vi "Memory.Pointer.Write.Safe.1D.U64.vi"(8 "error in (no error)":errorcluster, 9 "count":u64 format="%d elements", 10 "buffer in":u64[](array[numeric]), 11 "pointer in":refnum<class "Memory.Pointer.lvclass">) -> (0 "error out":errorcluster, 2 "buffer out":u64[](array[numeric]), 3 "pointer out":refnum<class "Memory.Pointer.lvclass">)   [LabVIEW 2016, in "Memory Manager.lvlib" / "Memory.Pointer.lvclass"]
doc: "Writes <b>count</b> elements from the provided <b>buffer</b> to the address specified by <b>pointer</b>.\n\n<b>Note:</b> This VI is <b>safe</b>.\n\nSafe means that this function evaluates the size parameter of <b>pointer</b> to ensure that is inbounds of allocated memory before peforming a memory read/write. Reading/writing more data to a pointer than it has allocated can corrupt or crash LabVIEW."
uses:
  Memory.Pointer.lvclass
  Memory.Pointer.lvclass/Memory.Pointer.ctl
  Accessors/Get Address.vi
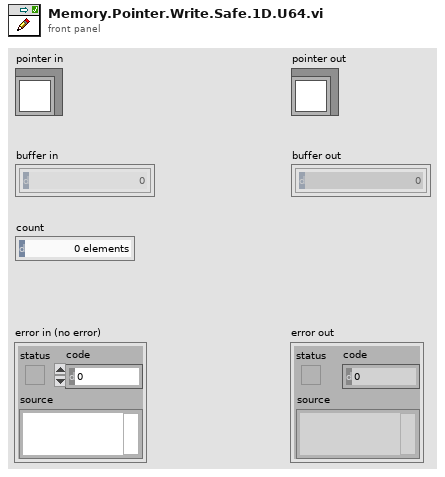
[diagram p1: front panel]
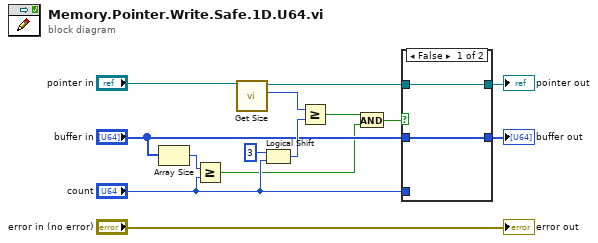
[diagram p0: block diagram]
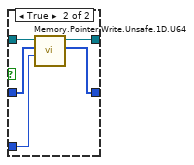
[diagram p2: hidden frame]
diagram:
  n1 = Array Size(array="buffer in") -> (size(s)=w3:i32)
  n2 = Greater Or Equal?(x=w3, y="count") -> (x >= y?=w1:bool)
  n3 = call "Get Size.vi"("Pointer in"="pointer in") -> ("size"=w7:u64, "Pointer out"=w12:refnum<class "Memory.Pointer.lvclass">)  [unwired: 8 in, 1 out]
  n4 = Logical Shift(y=i16 3, x="count") -> (x << y=w8:u64)
  n5 = Greater Or Equal?(x=w7, y=w8) -> (x >= y?=w5:bool)
  n6 = And(x=w5, y=w1) -> (x .and. y?=w6:bool)
  n7 = case shown="False" w6 {
    tunnel: w12 -> [w16 w21]
    tunnel: [w16 w20] -> w11
    tunnel: "buffer in" -> [w15 w19]
    tunnel: "count" -> [_ w18]
    tunnel: [w15 w17] -> w10
    frame False {
    }
    frame True {
      n8 = call "Memory.Pointer.Write.Unsafe.1D.U64.vi"("count"=w18, "buffer in"=w19, "pointer in"=w21) -> ("buffer out"=w17:u64[], "pointer out"=w20:refnum<class "Memory.Pointer.lvclass">)  [unwired: 6 in, 1 out]
    }
  }
  "pointer out" <- w11
  "buffer out" <- w10
  "error out" <- "error in (no error)"
